vi "Update AO AE.vi"(7 "Comm":enum16{"Init", "Read", "Write", "Close"}(ring), 8 "error in (no error)":errorcluster, 11 "AO Name":refnum<vi>) -> (0 "error out":errorcluster)   [LabVIEW 2016, in "DAQ Hardware.lvlib"]
uses:
  DAQ Hardware/DAQ Hardware.lvlib
panel:
  in  "Data In":dbl
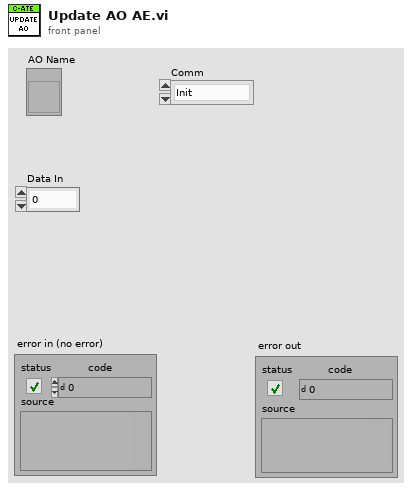
[diagram p1: front panel]
types:
  T1 = typedef "LVComboBoxStrsAndValuesArrayTypeDef.ctl" = cluster{"String":string, "Value":string}[]
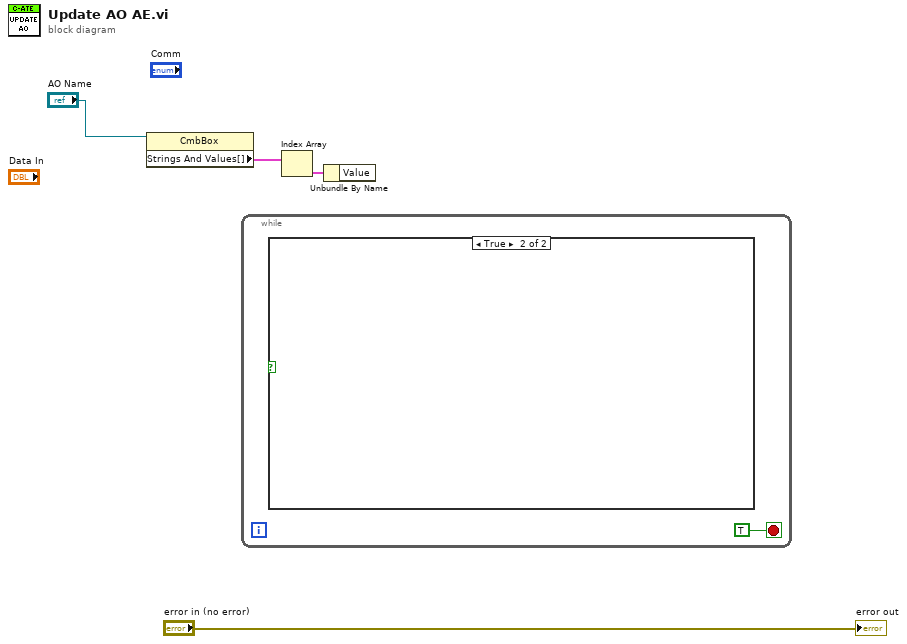
[diagram p0: block diagram]
diagram:
  n1 = property class="CmbBox"(reference="AO Name") -> ("Strings And Values[]"=w4:T1)  [unwired: 1 in, 2 out]
  n2 = while {
    stop <- TRUE stop-if-true
    n3 = case shown="True" {
      selector: _ -> [_ _]
      frame False {
      }
      frame True {
      }
    }
  }
  n4 = Index Array(array=w4) -> (element=w3:cluster{"String":string, "Value":string})  [unwired: 1 in]
  n5 = Unbundle By Name(w3) -> ()  [unwired: 1 out]
  "error out" <- "error in (no error)"
